vi "CRYSet Add Steps Front Panel.vi"(11 "Vi Ref":refnum<vi>) -> ()   [LabVIEW 2013]
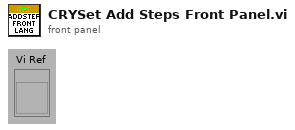
[diagram p1: front panel]
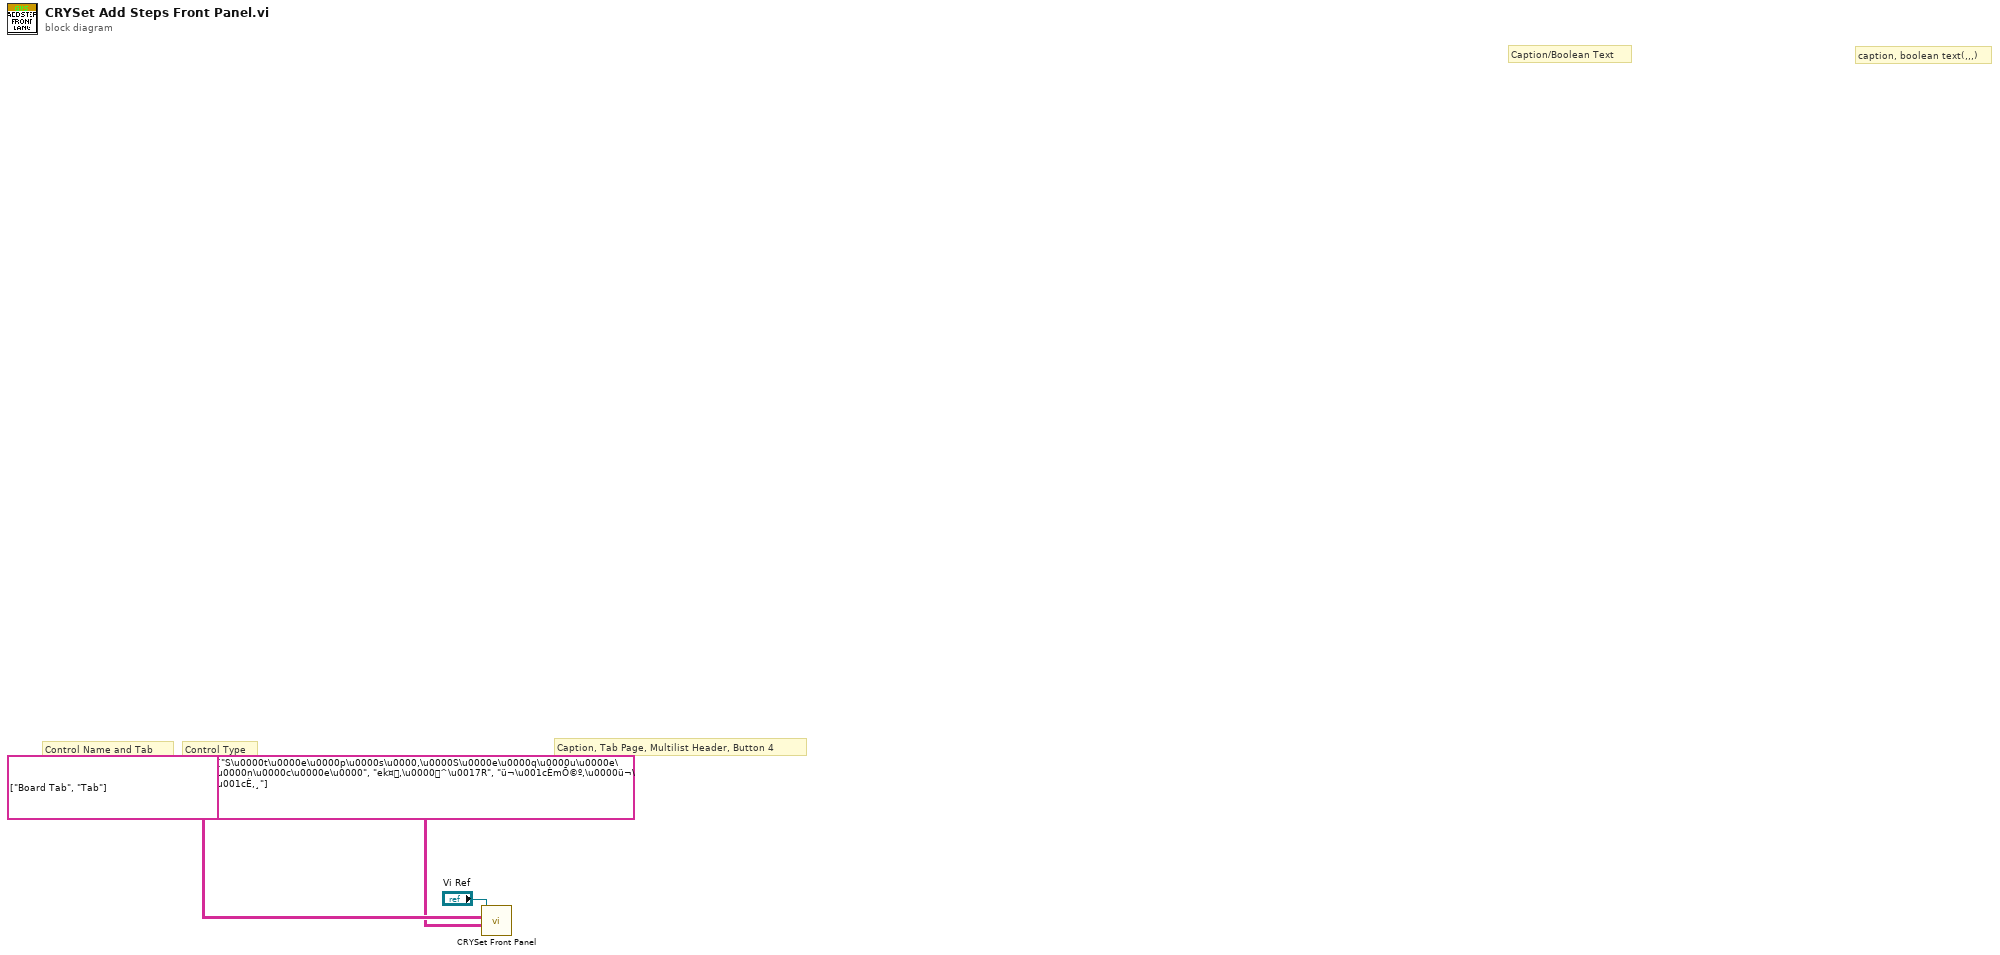
[diagram p0: block diagram]
diagram:
  # "Caption, Tab Page, Multilist Header, Button 4"
  # "Control Type"
  # "Control Name and Tab"
  # "caption, boolean text(,,,)"
  # "Caption/Boolean Text"
  n1 = call "CRYSet Front Panel.vi"("Caption(Boolean Text)"=string[][] [["S\u0000t\u0000e\u0000p\u0000s\u0000,\u0000S\u0000e\u0000q\u0000u\u0000e\u0000n\u0000c\u0000e\u0000", "ek¤,\u0000^\u0017R", "ü¬\u001cÈmÕ©º,\u0000ü¬\u001cÈ,¸"]], "Control ID and Type(Label Name, Type)"=string[][] [["Board Tab", "Tab"]], "Vi Ref"="Vi Ref") -> ()  [unwired: 9 in]
